vi "get.Ordered.FieldSpecs.vi"(8 "error in (no error)":errorcluster, 11 "PitchMessage in":refnum<class "PitchMessage.lvclass">) -> (0 "error out":errorcluster, 2 "orderedFieldSpecs":T1[](array[typedef]), 3 "PitchMessage out":refnum<class "PitchMessage.lvclass">)   [LabVIEW 2020, in "PitchMessage.lvclass"]
uses:
  PitchMessage.lvclass
  FieldSpec.ctl
  PitchMessage.lvclass/PitchMessage.ctl
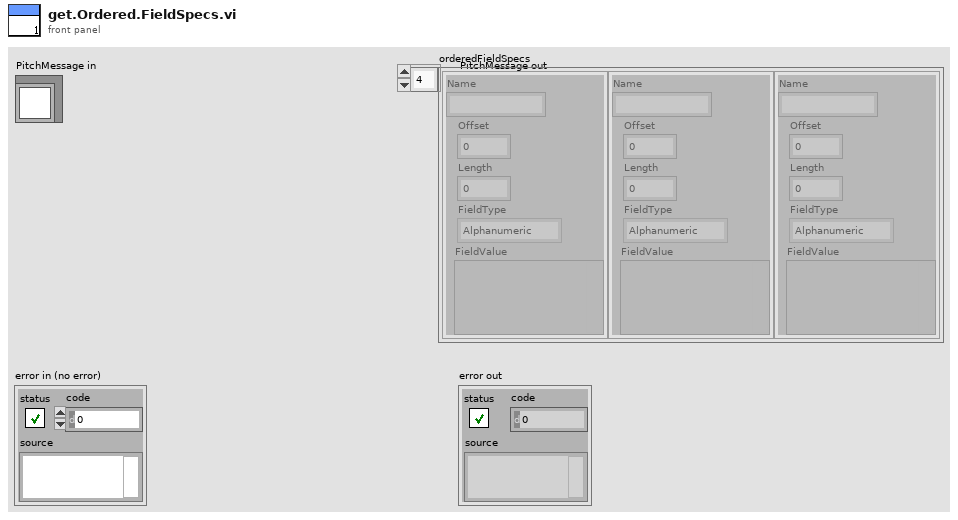
[diagram p1: front panel]
types:
  T1 = typedef "FieldSpec.ctl" = cluster{"Name":string, "Offset":i32, "Length":i32, "FieldType":enum16{"Alphanumeric", "Binary", "BinaryLongPrice", "BinaryShortPrice", "BitField", "PrintableAscii", "Value"}, "FieldValue":variant}
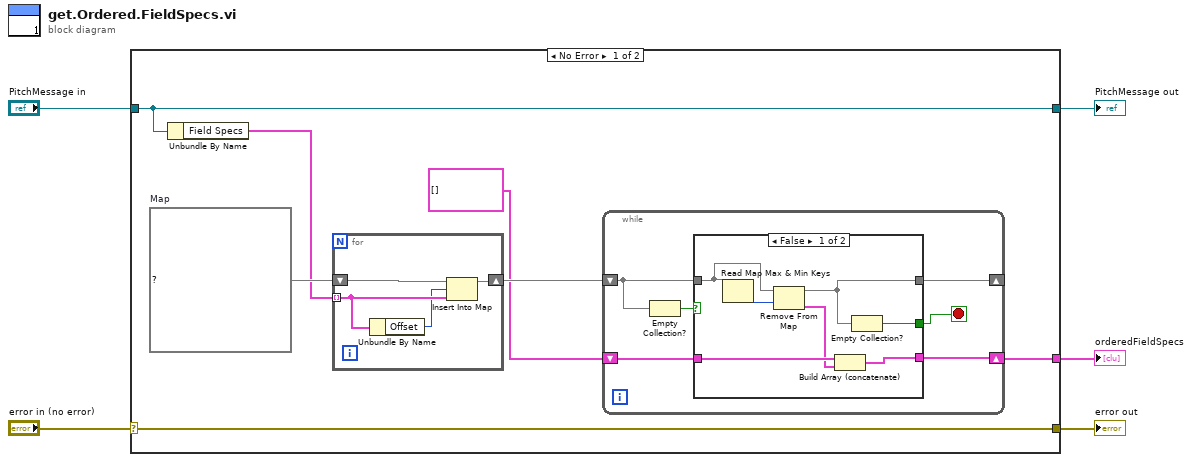
[diagram p0: block diagram]
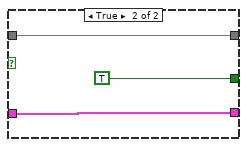
[diagram p2: hidden frame]
diagram:
  n1 = case shown="No Error" "error in (no error)" {
    selector: "error in (no error)" -> [w12 w34]
    tunnel: [w12 w34] -> w4
    tunnel: [w11 w33] -> w2
    tunnel: "PitchMessage in" -> [w11 w33]
    tunnel: [w6 _] -> w1
    frame No Error {
      w8 = map{i32, T1} {}  # Map
      n2 = Unbundle By Name(w11) -> ("Field Specs"=w7:T1[])
      n3 = for {
        tunnel: w7 -> [w31] mode=indexing
        shift-right: [w29] -> w10
        shift-left: w8 -> [w32]
        n4 = Unbundle By Name(w31) -> ("Offset"=w30:i32)
        n5 = Insert Into Map(map in=w32, key=w30, value=w31) -> (map out=w29:map{i32, T1})  [unwired: 2 out]
      }
      n6 = while {
        shift-right: [w16] -> _
        shift-left: w10 -> [w15]
        shift-right: [w14] -> w6
        shift-left: T1[] [] -> [w13]
        stop <- w17 stop-if-true
        n7 = Empty Collection?(1:w15) -> (0:w18:bool)
        n8 = case shown="False" w18 {
          tunnel: [w19 TRUE] -> w17
          tunnel: [w20 w27] -> w16
          tunnel: w15 -> [w22 w27]
          tunnel: [w24 w26] -> w14
          tunnel: w13 -> [w25 w26]
          frame False {
            n9 = Read Map Max & Min Keys(11:w22) -> (1:w23:i32)  [unwired: 1 out]
            n10 = Remove From Map(10:w23, 11:w22) -> (1:w21:T1, 3:w20:map{i32, T1})  [unwired: 1 out]
            n11 = Build Array (concatenate)(w25, w21) -> (w24:T1[])
            n12 = Empty Collection?(1:w20) -> (0:w19:bool)
          }
          frame True {
          }
        }
      }
    }
    frame Error {
    }
  }
  "error out" <- w4
  "PitchMessage out" <- w2
  "orderedFieldSpecs" <- w1
